vi "CAN Port Init.vi"(8 "error in (no error)":errorcluster, 10 "Selected Sockets":i16[](array[numeric]), 11 "ECU CAN Port":string) -> (0 "error out":errorcluster, 3 "CAN Ref Out":refnum<class "NI-XNET.lvclass">[](array[class]))   [LabVIEW 2023, in "LTT_TeststandSteptypes.lvlib"]
uses:
  LTT_TeststandSteptypes.lvlib
  HardwareAbstractionLayer_LVOOP/CAN/CAN Lib/NI-XNET_class/NI-XNET.lvclass
  Control/CAN FGV State.ctl
  HardwareAbstractionLayer_LVOOP/CAN/CAN Lib/CAN_class/Ctrls/CAN Init Ctrl.ctl
  <vilib>/xnet/xnet.llb/XNET Control Scope.ctl
  HardwareAbstractionLayer_LVOOP/CAN/CAN Lib/CAN_class/CAN.lvclass
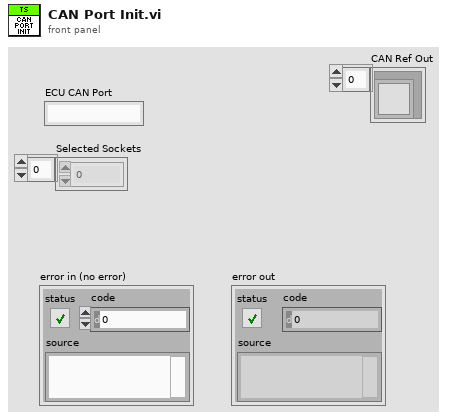
[diagram p1: front panel]
types:
  T1 = typedef "LTT_TeststandSteptypes.lvlib/CAN FGV State.ctl" = enum16{"Init", "Get", "Set"}
  T2 = typedef "HardwareAbstractionLayer_LVOOP.lvlib/CAN HAL Lib.lvlib/CAN.lvclass/CAN Init Ctrl.ctl" = cluster{"XNET Interface":refnum<k21>, "Baud Rate":u64, "CAN:Termination":u32, "Echo Transmit?":bool, "scope (normal)":T3}
  T3 = typedef "XNET Control Scope.ctl" = u32
  T4 = cluster{"Refnum out":refnum<k21>, "CAN Init Data":T2, "CAN_RxID":u32, "CAN_TxID":u32, "Timeout":dbl}
  T5 = typedef "LTT_TeststandSteptypes.lvlib/CAN Ref Data.ctl" = refnum<class "NI-XNET.lvclass">[]
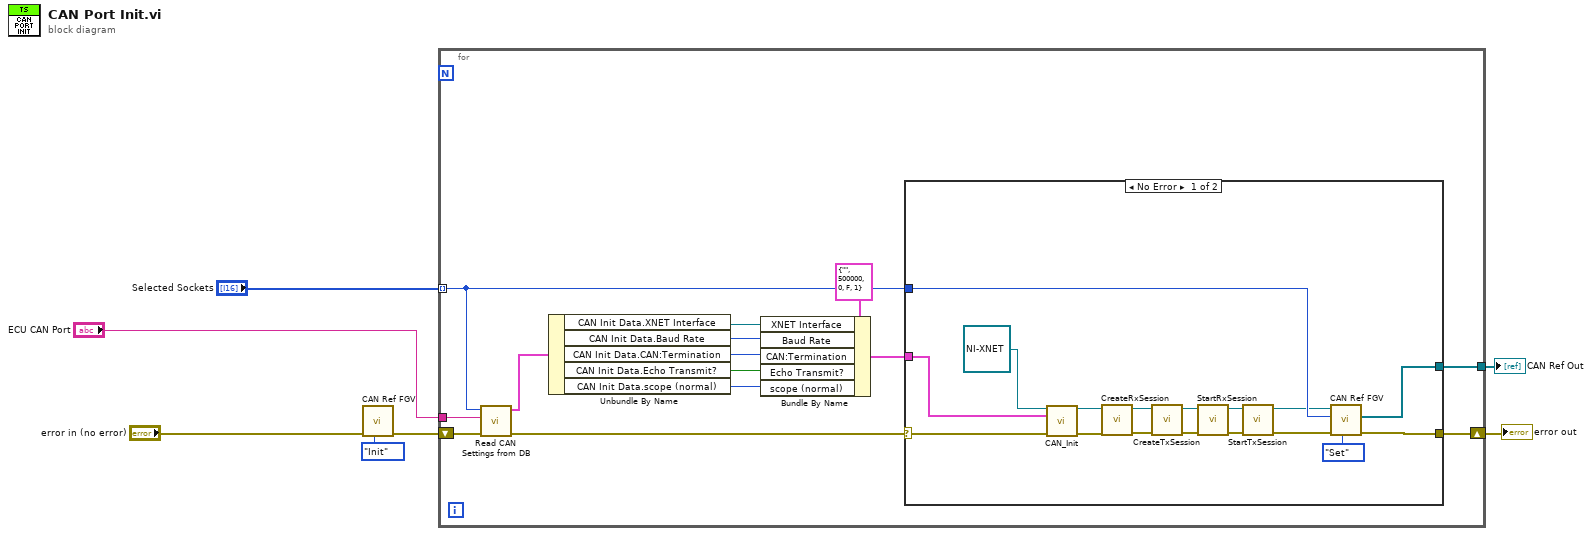
[diagram p0: block diagram]
diagram:
  n1 = call "CAN Ref FGV.vi"("CAN FGV State"=CAN_FGV_State."Init", "error in"="error in (no error)") -> ("error out"=w5:errorcluster)  [unwired: 7 in, 2 out]
  n2 = for {
    tunnel: "ECU CAN Port" -> [w19]
    shift-right: [w21] -> w2
    shift-left: w5 -> [w10]
    tunnel: "Selected Sockets" -> [w9] mode=indexing
    tunnel: [w8] -> w1
    n3 = call "Read CAN Settings from DB.vi"("error in"=w10, "ECU CAN Port"=w19, "Socket No"=w9) -> ("error out"=w20:errorcluster, "Read CAN Setting"=w16:T4)  [unwired: 7 in]
    n4 = Unbundle By Name(w16) -> ("CAN Init Data.XNET Interface"=w15:refnum<k21>, "CAN Init Data.Baud Rate"=w11:u64, "CAN Init Data.CAN:Termination"=w12:u32, "CAN Init Data.Echo Transmit?"=w13:bool, "CAN Init Data.scope (normal)"=w14:T3)
    n5 = Bundle By Name(cluster=T2 {"XNET Interface"="", "Baud Rate"=500000, "CAN:Termination"=0, "Echo Transmit?"=FALSE, "scope (normal)"=1} ("CAN Init Data"), "XNET Interface"=w15, "Baud Rate"=w11, "CAN:Termination"=w12, "Echo Transmit?"=w13, "scope (normal)"=w14) -> (w17:T2)
    n6 = case shown="No Error" w20 {
      selector: w20 -> [w30 w39]
      tunnel: [w26 w39] -> w21
      tunnel: w17 -> [w29 _]
      tunnel: w9 -> [w24 _]
      tunnel: [w22 _] -> w8
      frame No Error {
        n7 = call-dynamic "CAN_Init.vi"("object in"=refnum<class "NI-XNET.lvclass"> refnum, "CAN Init Data"=w29, "error in (no error)"=w30) -> ("object out"=w34:refnum<class "NI-XNET.lvclass">, "error out"=w33:errorcluster)  [unwired: 11 in]
        n8 = call-dynamic "CreateRxSession.vi"("error in (no error)"=w33, "NI-XNET in"=w34) -> ("error out"=w36:errorcluster, "NI-XNET out"=w35:refnum<class "NI-XNET.lvclass">)  [unwired: 8 in]
        n9 = call-dynamic "CreateTxSession.vi"("error in (no error)"=w36, "NI-XNET in"=w35) -> ("error out"=w31:errorcluster, "NI-XNET out"=w32:refnum<class "NI-XNET.lvclass">)  [unwired: 8 in]
        n10 = call-dynamic "StartRxSession.vi"("error in (no error)"=w31, "NI-XNET in"=w32) -> ("error out"=w38:errorcluster, "NI-XNET out"=w37:refnum<class "NI-XNET.lvclass">)  [unwired: 8 in]
        n11 = call-dynamic "StartTxSession.vi"("error in (no error)"=w38, "NI-XNET in"=w37) -> ("error out"=w27:errorcluster, "NI-XNET out"=w23:refnum<class "NI-XNET.lvclass">)  [unwired: 8 in]
        n12 = call "CAN Ref FGV.vi"("CAN FGV State"=CAN_FGV_State."Set", "error in"=w27, "Socket No"=w24, "object in"=w23) -> ("error out"=w26:errorcluster, "CAN Ref Data"=w22:T5)  [unwired: 5 in, 1 out]
      }
      frame Error {
      }
    }
  }
  "error out" <- w2
  "CAN Ref Out" <- w1
